vi "RefreshSubTree.vi"(8 "error in":errorcluster, 10 "node information":T1[](array[typedef]), 11 "tree ref in":refnum<vi>) -> (0 "error out":errorcluster, 3 "tree ref out":refnum<vi>)   [LabVIEW 2023, in "CEF.lvlib"]
doc: "Updates just a portion of the tree controlCopyright 2017 National Instruments Corporation\n\nLicensed under the Apache License, Version 2.0 (the \"License\"); you may not use this file except in compliance with the License. You may obtain a copy of the License at http://www.apache.org/licenses/LICENSE-2.0\nUnless required by applicable law or agreed to in writing, software distributed under the License is distributed on an \"AS IS\" BASIS, WITHOUT WARRANTIES OR CONDITIONS OF ANY KIND, either express or implied. See the License for the specific language governing permissions and limitations under the License."
uses:
  CEF.lvlib
  Node/Summary.ctl
  Node/CEF_Node.lvclass
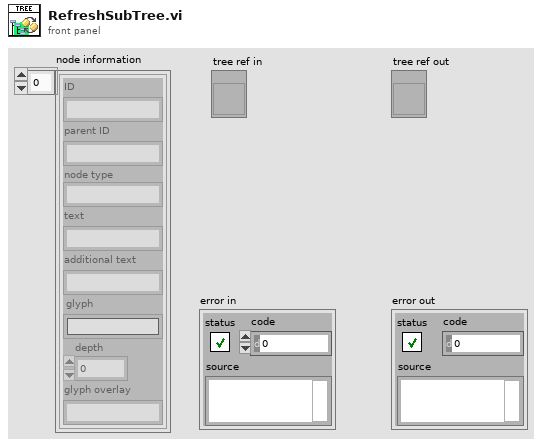
[diagram p1: front panel]
types:
  T1 = typedef "CEF.lvlib/CEF_Node.lvclass/Summary.ctl" = cluster{"ID":string, "parent ID":string, "node type":string, "text":string, "additional text":string, "glyph":string, "depth":i32, "glyph overlay":string}
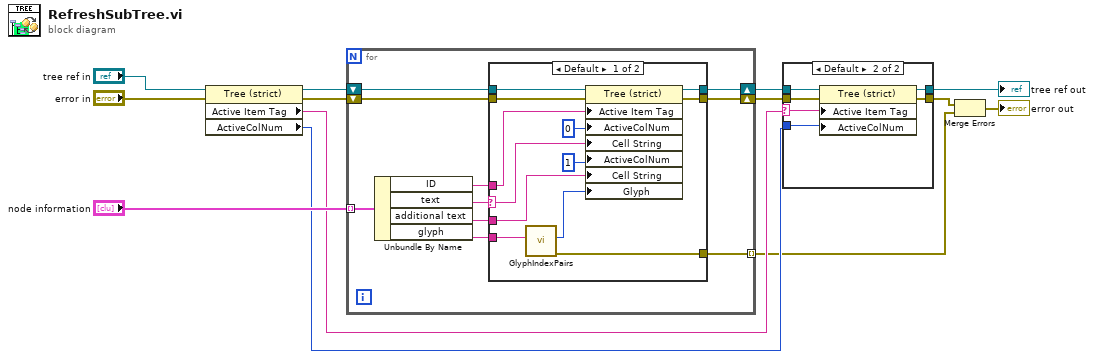
[diagram p0: block diagram]
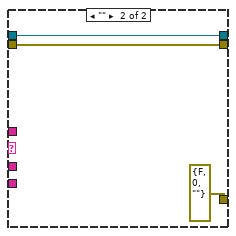
[diagram p3: hidden frame]
diagram:
  n1 = property class="Tree (strict)"(reference="tree ref in", error in="error in") -> (reference out=w11:refnum<vi>, error out=w9:errorcluster, "Active Item Tag"=w5:string, "ActiveColNum"=w4:i32)
  n2 = for {
    shift-right: [w22] -> w6
    shift-left: w9 -> [w21]
    tunnel: "node information" -> [w23] mode=indexing
    shift-right: [w19] -> w7
    shift-left: w11 -> [w18]
    tunnel: [w14] -> w2 mode=indexing
    n3 = Unbundle By Name(w23) -> ("ID"=w17:string, "text"=w20:string, "additional text"=w16:string, "glyph"=w15:string)
    n4 = case shown="Default" w20 {
      selector: w20 -> [w29 _]
      tunnel: [w32 w38] -> w22
      tunnel: w21 -> [w33 w38]
      tunnel: [w34 w37] -> w19
      tunnel: w18 -> [w35 w37]
      tunnel: w17 -> [w31 _]
      tunnel: w16 -> [w27 _]
      tunnel: w15 -> [w26 _]
      tunnel: [w24 errorcluster {"status"=FALSE, "code"=0, "source"=""} ("error out")] -> w14
      frame Default {
        n5 = call "GlyphIndexPairs.vi"("glyph"=w26) -> ("error out"=w24:errorcluster, "index"=w25:i32)  [unwired: 9 in]
        n6 = property class="Tree (strict)"(reference=w35, error in=w33, "Active Item Tag"=w31, "ActiveColNum"=0 ("Active Cell:Active Column Number"), "Cell String"=w29, "ActiveColNum"=1 ("Active Cell:Active Column Number"), "Cell String"=w27, "Glyph"=w25) -> (reference out=w34:refnum<vi>, error out=w32:errorcluster)
      }
      frame "" {
      }
    }
  }
  n7 = case shown="Default" w5 {
    selector: w5 -> [_ w41]
    tunnel: [w40 w46] -> w8
    tunnel: w7 -> [w40 w45]
    tunnel: w6 -> [w39 w44]
    tunnel: w4 -> [_ w43]
    tunnel: [w39 w42] -> w3
    frame "" {
    }
    frame Default {
      n8 = property class="Tree (strict)"(reference=w45, error in=w44, "Active Item Tag"=w41, "ActiveColNum"=w43) -> (reference out=w46:refnum<vi>, error out=w42:errorcluster)
    }
  }
  "tree ref out" <- w8
  n9 = Merge Errors(w3, w2) -> (→"error out":errorcluster)
